vi "ToTable.vi"(8 "error in":errorcluster, 9 "Table Index (0)":i32, 10 "variant":variant, 11 "PID Module 2 editor node in":refnum<class "PID Module 2 editor node.lvclass">) -> (0 "error out":errorcluster, 1 "row headers":string[](array[string]), 2 "table":string[][](array[string]), 3 "PID Module 2 editor node out":refnum<class "PID Module 2 editor node.lvclass">)   [LabVIEW 2015, in "PID Module 2 editor node.lvclass"]
doc: "Generates the strings needed to display on a table based on the information found in the engine and module configuration classes."
uses:
  PID Module 2 editor node.lvclass
  module/configuration/PID Module 2 configuration.lvclass
  <vilib>/NI/Module Execution Interface/Engine Configuration/engine configuration.lvclass
  module/configuration/PID Module 2 configuration.lvclass/PID Module 2 configuration.ctl
  <vilib>/NI/Configuration Framework/serializable configuration/NISE_CEF_serializable configuration.lvclass/NISE_CEF_serializable configuration.ctl
  module/configuration/Read Lines.vi
  <vilib>/Utility/LVClass/Get LV Class Name.vi
  <vilib>/NI/Configuration Framework/error generator/NISE_error generator.vi
  <vilib>/NI/Tag Bus Module Framework/channel/TBM channel.lvclass
  <vilib>/NI/Configuration Framework/serializable configuration/NISE_CEF_serializable configuration.lvclass
  <vilib>/NI/DCAF/Tag Editor Core/Table API/Table Manager.lvlib
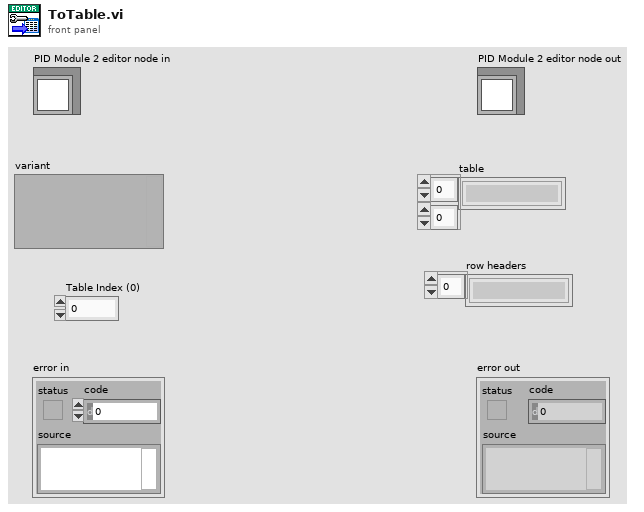
[diagram p1: front panel]
types:
  T1 = typedef "PID Module 2 configuration.lvclass/Line.ctl" = cluster{"PID ID":string, "Setpoint":refnum<class "TBM channel.lvclass">, "Variable":refnum<class "TBM channel.lvclass">, "Output":refnum<class "TBM channel.lvclass">, "Output High":refnum<class "TBM channel.lvclass">, "Output Low":refnum<class "TBM channel.lvclass">, "P":refnum<class "TBM channel.lvclass">, "I":refnum<class "TBM channel.lvclass">, "D":refnum<class "TBM channel.lvclass">}
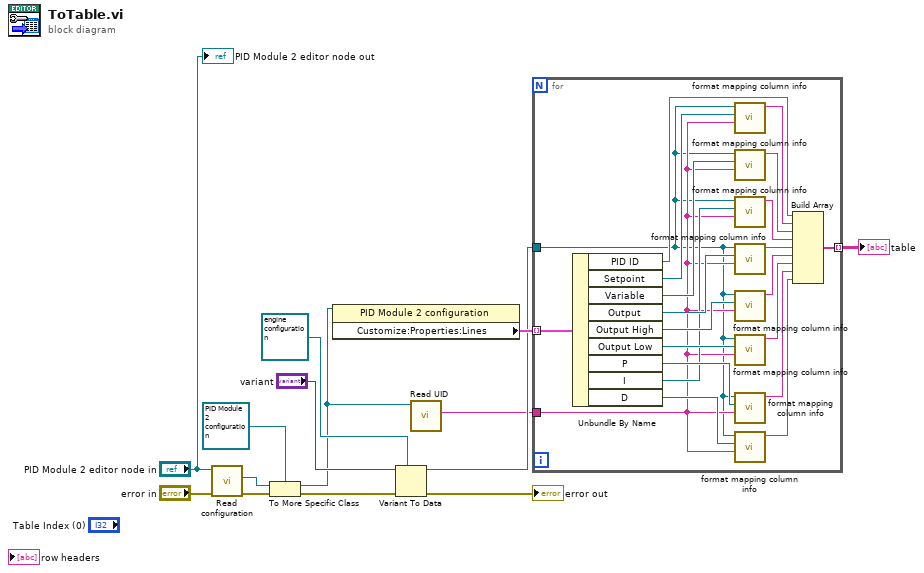
[diagram p0: block diagram]
diagram:
  n1 = call-dynamic "Read configuration.vi"("error in"="error in", "PID Module 2 editor node in"="PID Module 2 editor node in") -> ("error out"=w14:errorcluster, "configuration"=w5:refnum<class "NISE_CEF_serializable configuration.lvclass">)  [unwired: 7 in, 1 out]
  n2 = To More Specific Class(target class=refnum<class "PID Module 2 configuration.lvclass"> refnum ("tag bus configurable plugin module configuration"), reference=w5, error in=w14) -> (specific class reference=w4:refnum<class "PID Module 2 configuration.lvclass">, error out=w2:errorcluster)
  n3 = property class="PID Module 2 configuration"(reference=w4) -> ("Customize:Properties:Lines"=w11:T1[])  [unwired: 1 in, 2 out]
  n4 = Variant To Data(error in=w2, type=refnum<class "engine configuration.lvclass"> refnum ("engine configuration"), Variant="variant") -> (data=w8:refnum<class "engine configuration.lvclass">, error out=→"error out":errorcluster)
  n5 = call <vilib>:"Read UID.vi"("configuration in"=w4) -> ("instance id"=w3:string)  [unwired: 8 in, 2 out]
  n6 = for {
    tunnel: w11 -> [w35] mode=indexing
    tunnel: w8 -> [w15]
    tunnel: [w34] -> w6 mode=indexing
    tunnel: w3 -> [w24]
    n7 = Unbundle By Name(w35) -> ("PID ID"=w33:string, "Setpoint"=w32:refnum<class "TBM channel.lvclass">, "Variable"=w31:refnum<class "TBM channel.lvclass">, "Output"=w30:refnum<class "TBM channel.lvclass">, "Output High"=w29:refnum<class "TBM channel.lvclass">, "Output Low"=w28:refnum<class "TBM channel.lvclass">, "P"=w27:refnum<class "TBM channel.lvclass">, "I"=w26:refnum<class "TBM channel.lvclass">, "D"=w25:refnum<class "TBM channel.lvclass">)
    n8 = call <vilib>:"format mapping column info.vi"("instance id"=w24, "channel"=w32, "engine configuration in"=w15) -> ("mapping info"=w23:string)  [unwired: 8 in]
    n9 = call <vilib>:"format mapping column info.vi"("instance id"=w24, "channel"=w31, "engine configuration in"=w15) -> ("mapping info"=w22:string)  [unwired: 8 in]
    n10 = call <vilib>:"format mapping column info.vi"("instance id"=w24, "channel"=w26, "engine configuration in"=w15) -> ("mapping info"=w21:string)  [unwired: 8 in]
    n11 = call <vilib>:"format mapping column info.vi"("instance id"=w24, "channel"=w30, "engine configuration in"=w15) -> ("mapping info"=w20:string)  [unwired: 8 in]
    n12 = call <vilib>:"format mapping column info.vi"("instance id"=w24, "channel"=w29, "engine configuration in"=w15) -> ("mapping info"=w19:string)  [unwired: 8 in]
    n13 = call <vilib>:"format mapping column info.vi"("instance id"=w24, "channel"=w28, "engine configuration in"=w15) -> ("mapping info"=w18:string)  [unwired: 8 in]
    n14 = call <vilib>:"format mapping column info.vi"("instance id"=w24, "channel"=w27, "engine configuration in"=w15) -> ("mapping info"=w17:string)  [unwired: 8 in]
    n15 = call <vilib>:"format mapping column info.vi"("instance id"=w24, "channel"=w25, "engine configuration in"=w15) -> ("mapping info"=w16:string)  [unwired: 8 in]
    n16 = Build Array(w33, w23, w22, w21, w20, w19, w18, w17, w16) -> (w34:string[])
  }
  "table" <- w6
  "PID Module 2 editor node out" <- "PID Module 2 editor node in"
